vi "Mask VI.vi"(10 "y":dbl, 11 "x":dbl) -> (0 "Application:Version Year":string, 1 "Application:Version Number":string, 2 "Application:Name":string, 3 "x+y":dbl)   [LabVIEW 2019]
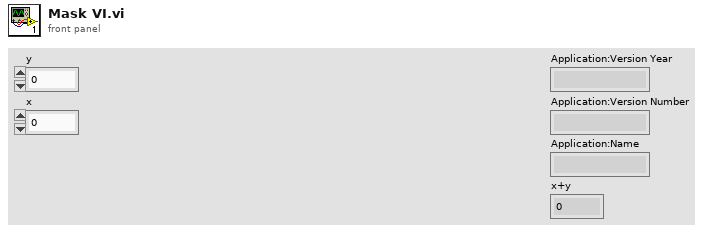
[diagram p1: front panel]
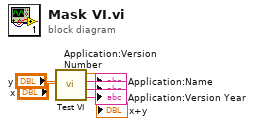
[diagram p0: block diagram]
diagram:
  n1 = call "Test VI.vi"("y"="y", "x"="x") -> ("Application:Version Year"=→"Application:Version Year":string, "Application:Version Number"=→"Application:Version Number":string, "Application:Name"=→"Application:Name":string, "x+y"=→"x+y":dbl)  [unwired: 5 in]
